vi "PH_gentec_Powermeter.get Information.vi"(0 "i ref in":refnum<vi>, 5 "error in":errorcluster) -> (13 "Timeout?":bool, 14 "i ref out":refnum<vi>, 17 "Error Messages":string, 18 "Device Error out":errorcluster, 19 "error out":errorcluster)   [LabVIEW 2014, in "PH_gentec_Powermeter.lvlib"]
doc: "This VI gets the basic information from the device, stores it at own attributes and indicates it at the GUI."
uses:
  PH_gentec_Powermeter.lvlib
  non_GPL/instr.lib/gentec-SOLO-PE/Driver/Type Defs/gentec-SOLO-PE.Scale.ctl
  PH_Powermeter_BaseClass/PH_gentec_BaseClass.Head Settings.ctl
  non_GPL/instr.lib/gentec-SOLO-PE/Driver/Type Defs/gentec-SOLO-PE.Queries with String Answers.ctl
  PH_gentec_Powermeter.Sets.ctl
  non_GPL/instr.lib/gentec-SOLO-PE/Driver/Type Defs/gentec-SOLO-PE.Data Sampling Settings.ctl
  PH_Powermeter_BaseClass/PH_Powermeter_BaseClass.Head Attributes.ctl
  PH_Powermeter_BaseClass/PH_Powermeter_BaseClass.lvlib
  non_GPL/instr.lib/gentec-SOLO-PE/gentec-SOLO-PE - Driver.lvlib
panel:
  in  "Dummy":T1 items=["Auto", "1 pJ", "3 pJ", "10 pJ", "30 pJ", "100 pJ", "300 pJ", "1 nJ", "3 nJ", "10 nJ", "30 nJ", "100 nJ", "300 nJ", "1 uJ", "3 uJ", "10 uJ", "30 uJ", "100 uJ", "300 uJ", "1 mJ", "3 mJ", "10 mJ", "30 mJ", "100 mJ", "300 mJ", "1 J", "3 J", "10 J", "30 J", "100 J", "300 J", "1 kJ", "3 kJ", "10 kJ", "30 kJ", "100 kJ", "300 kJ", "1 MJ", "3 MJ", "10 MJ", "30 MJ", "100 MJ", "300 MJ"]
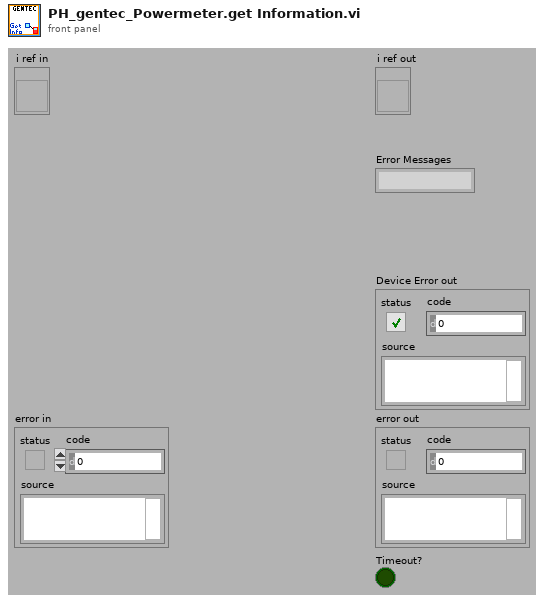
[diagram p1: front panel]
types:
  T1 = typedef "gentec-SOLO-PE - Driver.lvlib/gentec-SOLO-PE.Scale.ctl" = u32
  T2 = typedef "PH_Powermeter_BaseClass.lvlib/PH_Powermeter_BaseClass.Head Attributes.ctl" = cluster{"Instrument Type":string, "Head Version":string, "Head Name":string, "Serial Number":string, "Firmware":string, "Sensor Type":string, "MinimumRange":u32, "Maximum Range":u32, "Min Wavelength":i32, "Max Wavelength":i32}
  T3 = typedef "PH_gentec_Powermeter.lvlib/PH_gentec_Powermeter.Sets.ctl" = cluster{"Data Sampling Settings":T4, "Set Zero":bool}
  T4 = typedef "gentec-SOLO-PE - Driver.lvlib/gentec-SOLO-PE.Data Sampling Settings.ctl" = cluster{"Sample Rate":u32, "Sample Rate Unit":u32, "Sample Period":u32, "Sample Period Unit":u32, "Total Duration":u32, "Total Duration Unit":u32, "Time Stamp":u32}
  T5 = typedef "gentec-SOLO-PE - Driver.lvlib/gentec-SOLO-PE.Queries with String Answers.ctl" = string
  T6 = typedef "PH_Powermeter_BaseClass.lvlib/PH_gentec_BaseClass.Head Settings.ctl" = cluster{"Trigger Level":dbl, "Wavelength":u32, "Range":u32}
  T7 = typedef "PH_Powermeter_BaseClass.lvlib/PH_Powermeter_BaseClass.i attribute.ctl" = cluster{"GUI References":T8, "Connection":T9, "Head Attributes":T2, "VISA resource":refnum<visa-resource-name>, "Energy":T11, "Service ID Energy":i32, "Wanted Settings":T6, "Current Settings":T6}
  T8 = typedef "PH_Powermeter_BaseClass.lvlib/PH_Powermeter_BaseClass.GUI Refs.ctl" = cluster{"Head Attributes":refnum<vi>, "Energy":refnum<vi>, "Connection":refnum<vi>, "VISA Resource":refnum<vi>, "Energy evolution":refnum<vi>, "Scaling Factor":refnum<vi>, "Range":refnum<vi>, "Wavelength":refnum<vi>, "Trigger Level":refnum<vi>, "Wanted Settings":refnum<vi>, "Current Settings":refnum<vi>}
  T9 = typedef "PH_Powermeter_BaseClass.lvlib/PH_Powermeter_BaseClass.Connection.ctl" = cluster{"failed checks":i8, "Timeout":bool, "Data read":string, "Failure":bool, "Error":bool, "State":T10}
  T10 = typedef "PH_Powermeter_BaseClass.lvlib/PH_Powermeter_BaseClass.State.ctl" = enum32{"off", "operating", "opened", "checked", "connected", "Sets to change", "running"}
  T11 = typedef "PH_Powermeter_BaseClass.lvlib/PH_Powermeter_BaseClass.Energy.ctl" = cluster{"current Value":dbl, "unscaled":dbl, "Scaling Factor":dbl}
  T12 = typedef "gentec-SOLO-PE - Driver.lvlib/gentec-SOLO-PE.Configuration Values.ctl" = cluster{"Head Type":string, "Head Version":u32, "Serial Number":string, "Calibration Sensitivity":dbl, "Default Wavelength":u32, "Active Sensitivity":dbl, "Active Wavelength":u32, "Scale Min Power":u32, "Scale Max Power":u32, "Scale Min Energy":T1, "Scale Max Energy":T1, "Current Scale":T1, "Calo Mode":bool, "Anticipation":bool, "External Trig":bool, "Trig Level":dbl, "Zero Offset":dbl, "Multiplier 1":dbl, "Offset 1":dbl, "Multiplier 2":dbl, "Offset 2":dbl, "Max Power (Joulemeter)":dbl, "Max energy (Joulemeter)":dbl, "Currently Logging":bool, "Analog Out Active":bool, "Resolution":dbl, "Currently Calculating Stats":bool, "High-Resolution Display":bool, "Scale Min Wavelenght":u32, "Scale Max Wavelenght":u32, "Upper Bound":dbl, "Lower Bond":dbl, "Reference Value":dbl, "Thresholds Active":bool, "Fail":bool}
  T13 = typedef "LVStringsAndValuesArrayTypeDef_U32.ctl" = cluster{"String":string, "Value":u32}[]
  T14 = typedef "PH_gentec_Powermeter.lvlib/PH_gentec_Powermeter.i attribute.ctl" = cluster{"GUI References":cluster{"delete":refnum<vi>, "start stop Statistics":refnum<vi>, "Statistic Data":refnum<vi>, "Configuration Values":refnum<vi>, "Set Zero":refnum<vi>, "Data Sampling Settings":refnum<vi>, "Wanted Sets":refnum<vi>, "Current Sets":refnum<vi>}, "Start Stop Statistics":bool, "Wanted Sets":T3, "Current Sets":T3}
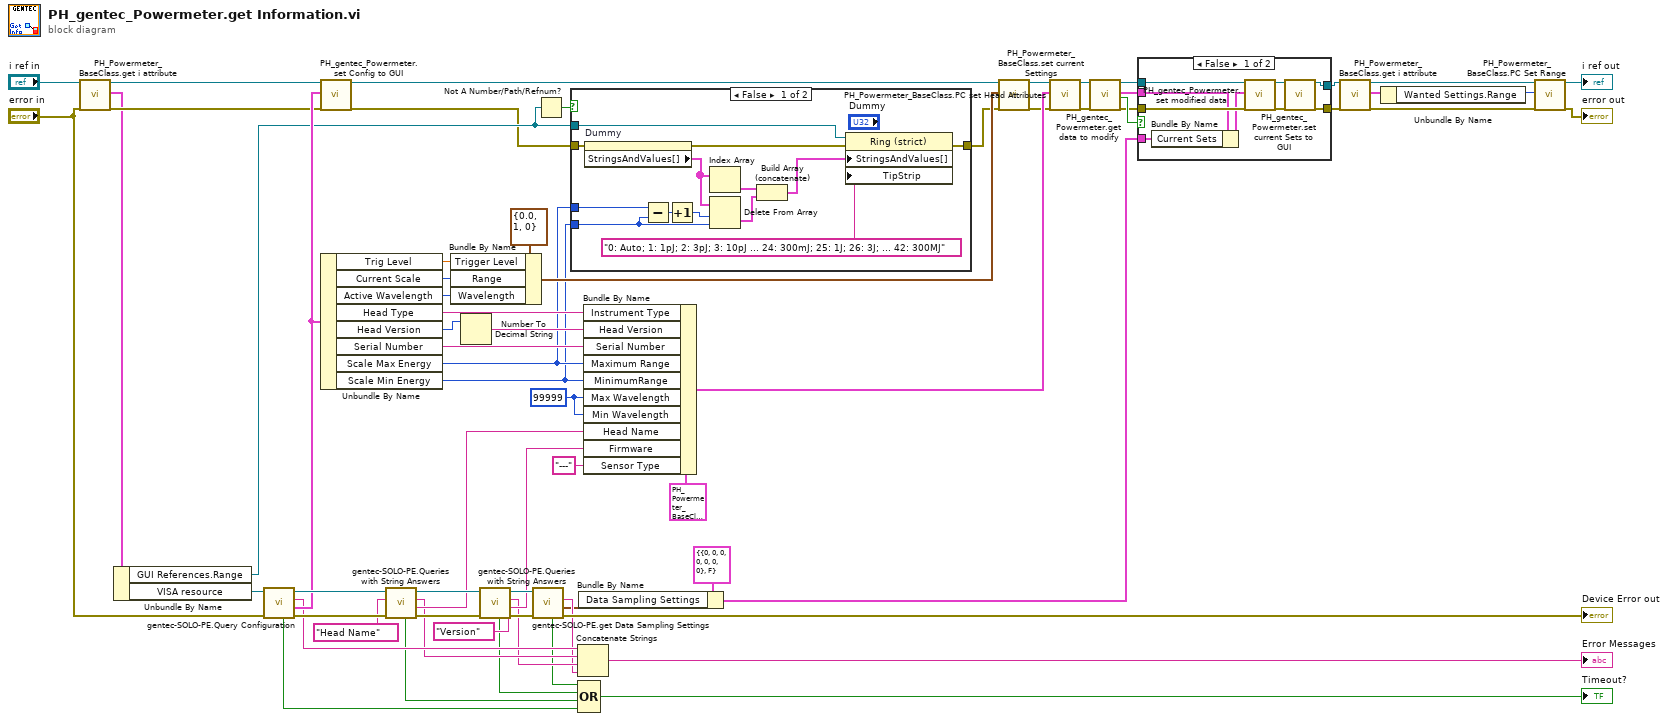
[diagram p0: block diagram]
diagram:
  w52 = 99999 ("Max Wavelength")
  n1 = call "PH_Powermeter_BaseClass.get i attribute.vi"("i ref in"="i ref in", "error in (no error)"="error in") -> ("i ref out"=w10:refnum<vi>, "i attribute"=w9:T7, "error out"=w12:errorcluster)  [unwired: 15 in]
  n2 = Unbundle By Name(w9) -> ("GUI References.Range"=w5:refnum<vi>, "VISA resource"=w7:refnum<visa-resource-name>)
  n3 = call "gentec-SOLO-PE.Query Configuration.vi"("error in (no error)"="error in", "VISA Refnum in"=w7) -> ("error out"=w54:errorcluster, "Configuration"=w49:T12, "Error"=w48:string, "VISA Refnum out"=w55:refnum<visa-resource-name>, "Timeout"=w38:bool)  [unwired: 5 in]
  n4 = call "PH_gentec_Powermeter.set Config to GUI.vi"("i ref in"=w10, "Configuration Values"=w49, "error in"=w12) -> ("i ref out"=w23:refnum<vi>, "error out"=w4:errorcluster)  [unwired: 15 in]
  n5 = Unbundle By Name(w49) -> ("Trig Level"=w22:dbl, "Current Scale"=w57:T1, "Active Wavelength"=w56:u32, "Head Type"=w53:string, "Head Version"=w65:u32, "Serial Number"=w66:string, "Scale Max Energy"=w2:T1, "Scale Min Energy"=w1:T1)
  n6 = call "gentec-SOLO-PE.Queries with String Answers.vi"("error in (no error)"=w54, "Queries with String Answers"=T5 "Head Name", "VISA Refnum in"=w55) -> ("error out"=w63:errorcluster, "Answer"=w47:string, "Error"=w45:string, "VISA Refnum out"=w62:refnum<visa-resource-name>, "Timeout"=w40:bool)  [unwired: 4 in]
  n7 = Bundle By Name(cluster=T6 {"Trigger Level"=0.0, "Wavelength"=1, "Range"=0} ("Current Settings"), "Trigger Level"=w22, "Range"=w57, "Wavelength"=w56) -> (w28:T6)
  n8 = Number To Decimal String(number=w65) -> (decimal integer string=w64:string)  [unwired: 1 in]
  n9 = call "gentec-SOLO-PE.Queries with String Answers.vi"("error in (no error)"=w63, "Queries with String Answers"=T5 "Version", "VISA Refnum in"=w62) -> ("error out"=w58:errorcluster, "Answer"=w46:string, "Error"=w44:string, "VISA Refnum out"=w59:refnum<visa-resource-name>, "Timeout"=w39:bool)  [unwired: 4 in]
  n10 = call "gentec-SOLO-PE.get Data Sampling Settings.vi"("error in (no error)"=w58, "VISA Refnum in"=w59) -> ("error out"=→"Device Error out":errorcluster, "Data Samling Settings"=w35:T4, "Error"=w43:string, "Timeout"=w41:bool)  [unwired: 5 in, 1 out]
  n11 = Not A Number/Path/Refnum?(number/path/refnum=w5) -> (NaN/Path/Refnum?=w6:bool)
  n12 = case shown="False" w6 {
    tunnel: [w80 w81] -> w3
    tunnel: w5 -> [w79 _]
    tunnel: w4 -> [w78 w81]
    tunnel: w2 -> [w70 _]
    tunnel: w1 -> [w69 _]
    frame False {
      n13 = property on="Dummy" class="Ring (strict)"(error in=w78) -> (error out=w77:errorcluster, "StringsAndValues[]"=w76:T13)  [unwired: 1 in, 1 out]
      n14 = Subtract(x=w70, y=w69) -> (x-y=w75:T1)
      n15 = Increment(x=w75) -> (x+1=w74:T1)
      n16 = Index Array(array=w76) -> (element=w73:cluster{"String":string, "Value":u32})  [unwired: 1 in]
      n17 = Delete From Array(array=w76, length=w74, index=w69) -> (deleted portion=w72:T13)  [unwired: 1 out]
      n18 = Build Array (concatenate)(w73, w72) -> (w71:T13)
      n19 = property class="Ring (strict)"(reference=w79, error in=w77, "StringsAndValues[]"=w71, "TipStrip"="0: Auto; 1: 1pJ; 2: 3pJ; 3: 10pJ ... 24: 300mJ; 25: 1J; 26: 3J; ... 42: 300MJ" ("Tip Strip")) -> (error out=w80:errorcluster)  [unwired: 1 out]
    }
    frame True {
    }
  }
  n20 = Concatenate Strings(w48, w45, w44, w43) -> (→"Error Messages":string)
  n21 = Compound Arithmetic op=OR(w41, w39, w40, w38) -> (→"Timeout?":bool)
  n22 = Bundle By Name(cluster=T3 {"Data Sampling Settings"={"Sample Rate"=0, "Sample Rate Unit"=0, "Sample Period"=0, "Sample Period Unit"=0, "Total Duration"=0, "Total Duration Unit"=0, "Time Stamp"=0}, "Set Zero"=FALSE} ("Current Sets"), "Data Sampling Settings"=w35) -> (w34:T3)
  n23 = Bundle By Name(cluster=T2 {"Instrument Type"="---", "Head Version"="---", "Head Name"="---", "Serial Number"="---", "Firmware"="---", "Sensor Type"="---", "MinimumRange"=0, "Maximum Range"=0, "Min Wavelength"=-1, "Max Wavelength"=-1} ("Head Attributes"), "Instrument Type"=w53, "Head Version"=w64, "Serial Number"=w66, "Maximum Range"=w2, "MinimumRange"=w1, "Max Wavelength"=w52, "Min Wavelength"=w52, "Head Name"=w47, "Firmware"=w46, "Sensor Type"="---" ("Head Name")) -> (w67:T2)
  n24 = call "PH_Powermeter_BaseClass.set current Settings.vi"("VI in"=w23, "Current Settings"=w28, "error in (no error)"=w3) -> ("VI out"=w27:refnum<vi>, "error out"=w26:errorcluster)  [unwired: 15 in]
  n25 = call "PH_Powermeter_BaseClass.PC set Head Attributes.vi"("VI in"=w27, "Head Attributes"=w67, "error in (no error)"=w26) -> ("VI out"=w25:refnum<vi>, "error out"=w13:errorcluster)  [unwired: 15 in]
  n26 = call "PH_gentec_Powermeter.get data to modify.vi"("i ref in"=w25, "error in (no error)"=w13) -> ("i ref out"=w30:refnum<vi>, "i attribute"=w31:T14, "timed out"=w32:bool, "error out"=w29:errorcluster)  [unwired: 14 in]
  n27 = case shown="False" w32 {
    tunnel: [w83 w92] -> w21
    tunnel: [w82 w91] -> w20
    tunnel: w29 -> [w89 w91]
    tunnel: w30 -> [w90 w92]
    tunnel: w31 -> [w88 _]
    tunnel: w34 -> [w86 _]
    frame False {
      n28 = Bundle By Name(cluster=w88, "Current Sets"=w86) -> (w87:T14)
      n29 = call "PH_gentec_Powermeter.set modified data.vi"("i ref in"=w90, "i attribute"=w87, "error in (no error)"=w89) -> ("i ref out"=w84:refnum<vi>, "error out"=w85:errorcluster)  [unwired: 15 in]
      n30 = call "PH_gentec_Powermeter.set current Sets to GUI.vi"("i ref in"=w84, "error in"=w85) -> ("i ref out"=w83:refnum<vi>, "error out"=w82:errorcluster)  [unwired: 16 in]
    }
    frame True {
    }
  }
  n31 = call "PH_Powermeter_BaseClass.get i attribute.vi"("i ref in"=w21, "error in (no error)"=w20) -> ("i ref out"=w18:refnum<vi>, "i attribute"=w17:T7, "error out"=w19:errorcluster)  [unwired: 15 in]
  n32 = Unbundle By Name(w17) -> ("Wanted Settings.Range"=w16:u32)
  n33 = call "PH_Powermeter_BaseClass.PC Set Range.vi"("VI in"=w18, "Wanted Range"=w16, "error in (no error)"=w19) -> ("VI out"=→"i ref out":refnum<vi>, "error out"=→"error out":errorcluster)  [unwired: 15 in]
